vi "Sub_InitChannels.vi"(2 "Channel_Series":T1 {"Switch Rate/s" format="%#_13g"}, 3 "Obj_Keithley":T2) -> (0 "Error Out":errorcluster, 1 "Keithley Out":refnum<visa-resource-name>)   [LabVIEW 2014]
uses:
  <vilib>/Instr/_visa.llb/VISA Configure Serial Port (Instr).vi
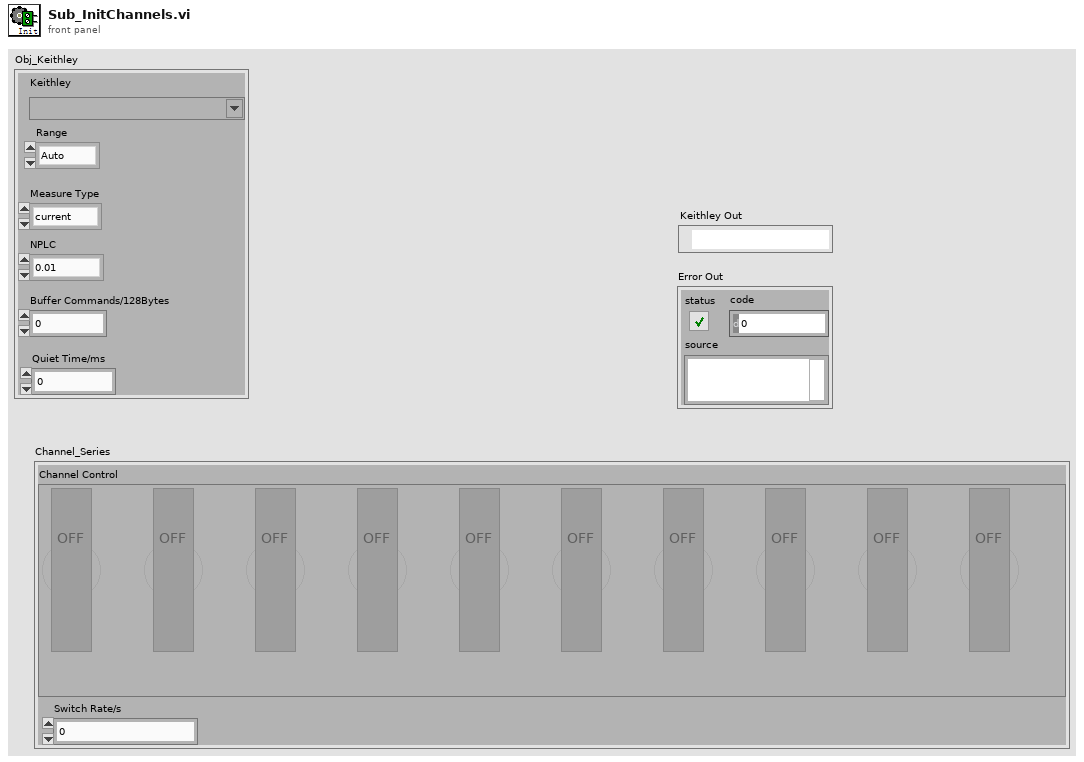
[diagram p1: front panel]
types:
  T1 = cluster{"Channel Control":bool[], "Switch Rate/s":dbl}
  T2 = cluster{"Measure Type":enum16{"current", "voltage", "resistance", "charge", ""}, "NPLC":enum16{"0.01", "0.1", "1"}, "Keithley":refnum<visa-resource-name>, "Range":enum16{"Auto", "1e-1", "1e-2", "1e-3", "1e-4", "1e-5", "1e-6", "1e-7", "1e-8"}, "Buffer Commands/128Bytes":i32, "Quiet Time/ms":i32}
  T3 = enum16{"current", "voltage", "resistance", "charge", ""}
  T4 = enum16{"Auto", "1e-1", "1e-2", "1e-3", "1e-4", "1e-5", "1e-6", "1e-7", "1e-8"}
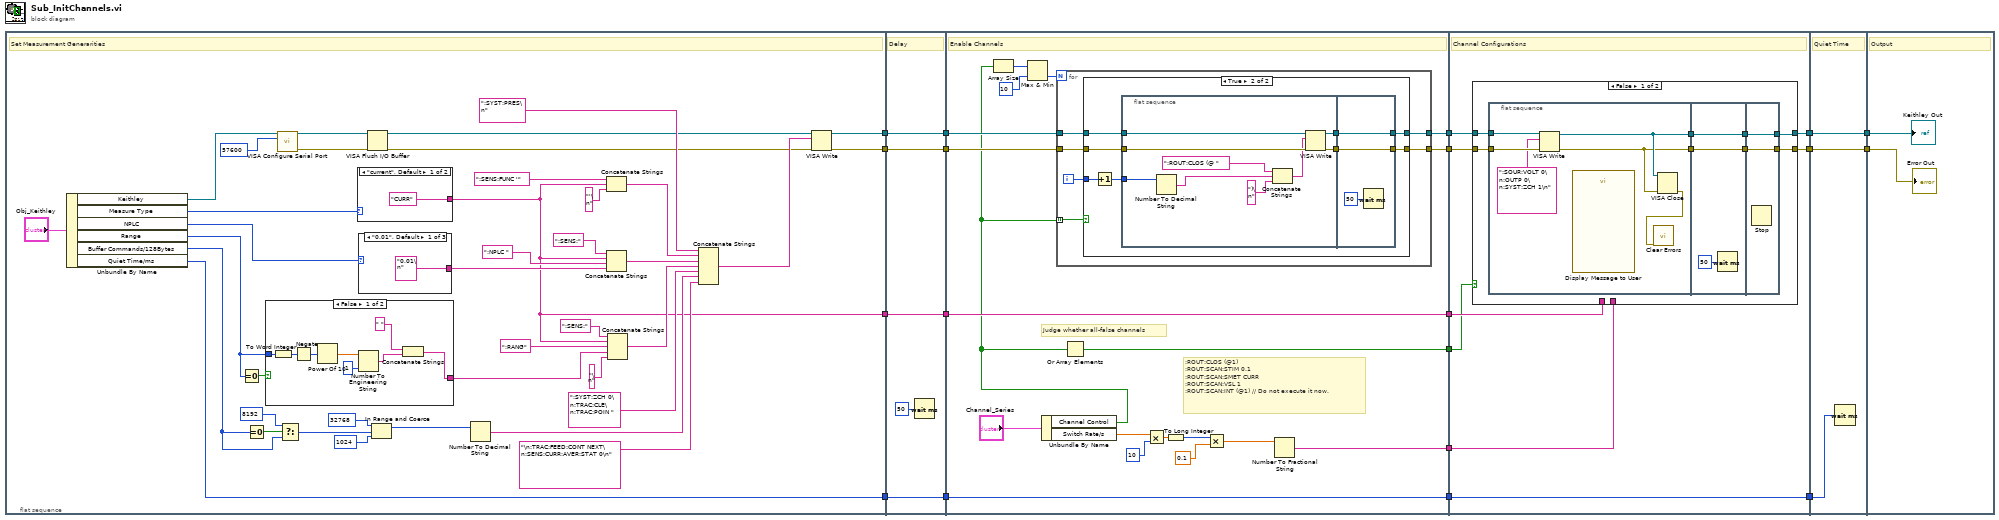
[diagram p0: block diagram]
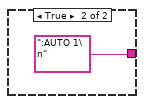
[diagram p2: hidden frame]
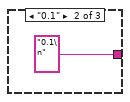
[diagram p3: hidden frame]
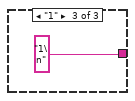
[diagram p4: hidden frame]
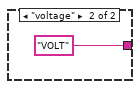
[diagram p5: hidden frame]
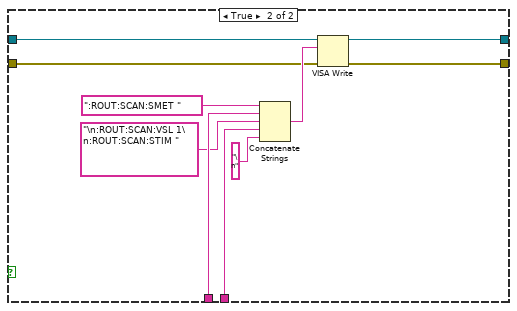
[diagram p7: hidden frame]
diagram:
  n1 = flat-sequence {
    tunnel: [w58] -> w19
    tunnel: [w57] -> w18
    tunnel: [w30] -> w14
    tunnel: [w29] -> w3
    tunnel: w19 -> [w76]
    tunnel: w18 -> [w75]
    tunnel: [w76] -> w17
    tunnel: [w75] -> w16
    tunnel: [w74] -> w15
    tunnel: w14 -> [w74]
    tunnel: [w73] -> w4
    tunnel: w3 -> [w73]
    tunnel: w17 -> [w95]
    tunnel: w16 -> [w94]
    tunnel: w15 -> [w88]
    tunnel: [w88] -> w13
    tunnel: [w87] -> w12
    tunnel: [w86] -> w11
    tunnel: [w84] -> w10
    tunnel: [w83] -> w9
    tunnel: w4 -> [w78]
    tunnel: [w78] -> w2
    tunnel: w13 -> [w131]
    tunnel: w12 -> [w132]
    tunnel: w11 -> [w130]
    tunnel: w10 -> [w129]
    tunnel: w9 -> [w128]
    tunnel: [w127] -> w8
    tunnel: [w126] -> w6
    tunnel: w2 -> [w125]
    tunnel: [w125] -> w1
    tunnel: w8 -> [w164]
    tunnel: [w164] -> w7
    tunnel: w6 -> [w163]
    tunnel: [w163] -> w5
    tunnel: w1 -> [w162]
    tunnel: w7 -> [w166]
    tunnel: w5 -> [w165]
    frame #0 {
      # "Set Measurement Generarities"
      n2 = Unbundle By Name("Obj_Keithley") -> ("Keithley"=w47:refnum<visa-resource-name>, "Measure Type"=w53:T3, "NPLC"=w52:enum16{"0.01", "0.1", "1"}, "Range"=w44:T4, "Buffer Commands/128Bytes"=w22:i32, "Quiet Time/ms"=w29:i32)
      n3 = Equal To 0?(x=w44) -> (x = 0?=w45:bool)
      n4 = Equal To 0?(x=w22) -> (x = 0?=w24:bool)
      n5 = case shown="False" w45 {
        tunnel: [w59 ":AUTO 1\n"] -> w40
        tunnel: w44 -> [w66 _]
        frame False {
          n6 = To Word Integer(number=w66) -> (16bit integer=w65:i16)
          n7 = Negate(x=w65) -> (-x=w64:i16)
          n8 = Power Of 10(x=w64) -> (10^x=w63:dbl)
          n9 = Number To Engineering String(2:i16 1 ("precision (6)"), 4:w63) -> (0:w60:string)  [unwired: 2 in]
          n10 = Concatenate Strings(" " ("string"), w60) -> (w59:string)
        }
        frame True {
        }
      }
      n11 = call-poly "VISA Configure Serial Port"("VISA resource name"=w47, "baud rate (9600)"=u32 57600) -> ("VISA resource name out"=w28:refnum<visa-resource-name>, "error out"=w27:errorcluster)  [unwired: 12 in]
      n12 = Select(t=8192 ("upper limit"), s=w24, f=w22) -> (s? t:f=w21:i32)
      n13 = case shown="\"current\", Default" w53 {
        tunnel: ["CURR" "VOLT"] -> w30
        frame "current", Default {
        }
        frame "voltage" {
        }
      }
      n14 = case shown="\"0.01\", Default" w52 {
        tunnel: ["0.01\n" "0.1\n" "1\n"] -> w48
        frame "0.01", Default {
        }
        frame "0.1" {
        }
        frame "1" {
        }
      }
      n15 = VISA Flush I/O Buffer(VISA resource name=w28, error in (no error)=w27) -> (VISA resource name out=w26:refnum<visa-resource-name>, error out=w25:errorcluster)  [unwired: 1 in]
      n16 = In Range and Coerce(upper limit=32768, x=w21, lower limit=1024) -> (coerced(x)=w20:i32)  [unwired: 1 out]
      n17 = Number To Decimal String(number=w20) -> (decimal integer string=w33:string)  [unwired: 1 in]
      n18 = Concatenate Strings(":SENS:FUNC '" ("string"), w30, "'\n" ("string")) -> (w39:string)
      n19 = Concatenate Strings(":SENS:" ("string"), w30, ":NPLC " ("string"), w48) -> (w38:string)
      n20 = Concatenate Strings(":SENS:" ("string"), w30, ":RANG" ("string"), w40, "\n" ("string")) -> (w37:string)
      n21 = Concatenate Strings(":SYST:PRES\n" ("string"), w39, w38, w37, ":SYST:ZCH 0\n:TRAC:CLE\n:TRAC:POIN " ("string"), w33, "\n:TRAC:FEED:CONT NEXT\n:SENS:CURR:AVER:STAT 0\n" ("string")) -> (w56:string)
      n22 = VISA Write(VISA resource name=w26, write buffer=w56, error in (no error)=w25) -> (VISA resource name out=w58:refnum<visa-resource-name>, error out=w57:errorcluster)  [unwired: 1 out]
    }
    frame #1 {
      # "Delay"
      n23 = Wait (ms)(milliseconds to wait=u32 50) -> ()  [unwired: 1 out]
    }
    frame #2 {
      # ":ROUT:CLOS (@1)\n:ROUT:SCAN:STIM 0.1\n:ROUT:SCAN:SMET CURR\n:ROUT:SCAN:VSL 1\n:ROUT:SCAN:INT (@1) // Do not execute it now."
      # "Judge whether all-false channels"
      # "Enable Channels"
      n24 = Unbundle By Name("Channel_Series") -> ("Channel Control"=w81:bool[], "Switch Rate/s"=w93:dbl)
      n25 = Array Size(array=w81) -> (size(s)=w80:i32)
      n26 = Max & Min(x=w80, y=10) -> (min(x,y)=w82:i32)  [unwired: 1 out]
      n27 = for {
        N: w82 -> [_]
        tunnel: w81 -> [w101] mode=indexing
        tunnel: w95 -> [w100]
        tunnel: w94 -> [w99]
        tunnel: [w98] -> w87
        tunnel: [w97] -> w86
        i -> [w102]
        n28 = case shown="True" w101 {
          tunnel: w102 -> [_ w112]
          tunnel: w100 -> [w104 w111]
          tunnel: w99 -> [w103 w110]
          tunnel: [w104 w106] -> w98
          tunnel: [w103 w105] -> w97
          frame False {
          }
          frame True {
            n29 = Increment(x=w112) -> (x+1=w109:i32)
            n30 = flat-sequence {
              tunnel: w111 -> [w121]
              tunnel: w110 -> [w120]
              tunnel: w109 -> [w116]
              tunnel: [w119] -> w108
              tunnel: [w118] -> w107
              tunnel: w108 -> [w123]
              tunnel: w107 -> [w122]
              tunnel: [w123] -> w106
              tunnel: [w122] -> w105
              frame #0 {
                n31 = Number To Decimal String(number=w116) -> (decimal integer string=w115:string)  [unwired: 1 in]
                n32 = Concatenate Strings(":ROUT:CLOS (@ " ("string"), w115, ")\n" ("string")) -> (w114:string)
                n33 = VISA Write(VISA resource name=w121, write buffer=w114, error in (no error)=w120) -> (VISA resource name out=w119:refnum<visa-resource-name>, error out=w118:errorcluster)  [unwired: 1 out]
              }
              frame #1 {
                n34 = Wait (ms)(milliseconds to wait=u32 50) -> ()  [unwired: 1 out]
              }
            }
          }
        }
      }
      n35 = Or Array Elements(Boolean array=w81) -> (logical OR=w83:bool)
      n36 = Multiply(x=w93, y=10) -> (x*y=w91:dbl)
      n37 = To Long Integer(number=w91) -> (32bit integer=w90:i32)
      n38 = Multiply(x=w90, y=0.1) -> (x*y=w85:dbl)
      n39 = Number To Fractional String(number=w85) -> (F-format string=w84:string)  [unwired: 3 in]
    }
    frame #3 {
      # "Channel Configurations"
      n40 = case shown="False" w128 {
        tunnel: w132 -> [w140 w161]
        tunnel: w131 -> [_ w159]
        tunnel: w130 -> [w139 w156]
        tunnel: w129 -> [_ w155]
        tunnel: [w138 w153] -> w127
        tunnel: [w137 w152] -> w126
        frame False {
          n41 = flat-sequence {
            tunnel: w140 -> [w146]
            tunnel: w139 -> [w145]
            tunnel: [w143] -> w136
            tunnel: [w142] -> w134
            tunnel: w136 -> [w149]
            tunnel: [w149] -> w135
            tunnel: w134 -> [w148]
            tunnel: [w148] -> w133
            tunnel: w135 -> [w151]
            tunnel: [w151] -> w138
            tunnel: [w150] -> w137
            tunnel: w133 -> [w150]
            frame #0 {
              n42 = VISA Write(VISA resource name=w146, write buffer=":SOUR:VOLT 0\n:OUTP 0\n:SYST:ZCH 1\n", error in (no error)=w145) -> (VISA resource name out=w143:refnum<visa-resource-name>, error out=w142:errorcluster)  [unwired: 1 out]
              n43 = call "Display Message to User"() -> ()  [unwired: 10 in, 2 out]
              n44 = VISA Close(VISA resource name=w143, error in (no error)=w142) -> (error out=w141:errorcluster)
              n45 = call <vilib>:"Clear Errors.vi"("error in (no error)"=w141) -> ()  [unwired: 5 in, 2 out]
            }
            frame #1 {
              n46 = Wait (ms)(milliseconds to wait=u32 50) -> ()  [unwired: 1 out]
            }
            frame #2 {
              n47 = Stop() -> ()  [unwired: 1 in]
            }
          }
        }
        frame True {
          n48 = Concatenate Strings(":ROUT:SCAN:SMET " ("string"), w159, "\n:ROUT:SCAN:VSL 1\n:ROUT:SCAN:STIM " ("string"), w155, "\n" ("string")) -> (w157:string)
          n49 = VISA Write(VISA resource name=w161, write buffer=w157, error in (no error)=w156) -> (VISA resource name out=w153:refnum<visa-resource-name>, error out=w152:errorcluster)  [unwired: 1 out]
        }
      }
    }
    frame #4 {
      # "Quiet Time"
      n50 = Wait (ms)(milliseconds to wait=w162) -> ()  [unwired: 1 out]
    }
    frame #5 {
      # "Output"
      "Keithley Out" <- w166
      "Error Out" <- w165
    }
  }
